vi "test_GetChipSize.vi"() -> ()   [LabVIEW 2023]
uses:
  <vilib>/addons/_JKI Toolkits/Caraya/classes/Assert/Assert Equal Value and Type_Variant.vi
  <vilib>/addons/_JKI Toolkits/Caraya/classes/Test/Test.lvclass
  <vilib>/addons/_JKI Toolkits/Caraya/classes/Assert/Assert.lvclass
  GenericDevice.lvclass
panel:
  out "Data":i32
  out "error out":errorcluster
  # "Locals"
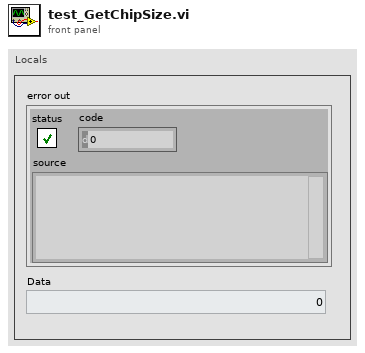
[diagram p1: front panel]
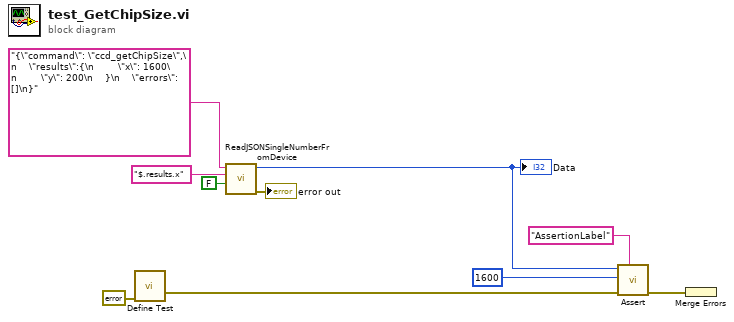
[diagram p0: block diagram]
diagram:
  n1 = call <vilib>:"Define Test.vi"("error in (no error)"=errorcluster {"status"=FALSE, "code"=0, "source"=""}) -> ("error out"=w4:errorcluster)  [unwired: 9 in, 1 out]
  n2 = call "ReadJSONSingleNumberFromDevice.vi"("timed out?"=FALSE, "JSON Key of Interest"="$.results.x" ("$Path or Item Name"), "JSON reply"="{\"command\": \"ccd_getChipSize\",\n    \"results\":{\n        \"x\": 1600\n        \"y\": 200\n    }\n    \"errors\": []\n}") -> ("error out"=→"error out":errorcluster, "Data"=w2:i32)  [unwired: 6 in, 1 out]
  "Data" <- w2
  n3 = call-poly <vilib>:"Assert.vi"("Label"="AssertionLabel" ("Label (VI Title)"), "error in (no error)"=w4, "Y"=1600 ("Data"), "X"=w2) -> ("error out"=w5:errorcluster)  [unwired: 6 in, 1 out]
  n4 = Merge Errors(w5) -> ()  [unwired: 1 out]
